vi "Create Summary Row.vi"(8 "error in (no error)":errorcluster, 10 "value":dbl, 11 "ACNET Device.lvclass":refnum<class "ACNET Device.lvclass">) -> (0 "error out":errorcluster, 3 "Summary Row":string[](array[string]))   [LabVIEW 2013, in "ACNET Monitor.lvlib"]
uses:
  ACNET Monitor.lvlib
  ACNET Device.lvclass
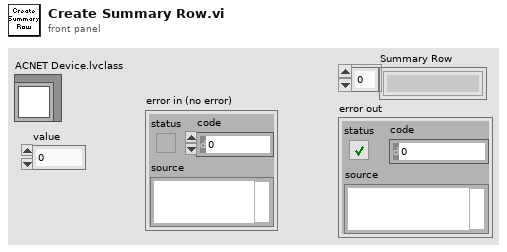
[diagram p1: front panel]
types:
  T1 = cluster{"name":string, "minValue":dbl, "maxValue":dbl, "units":string, "description":string, "ignoreMinValue":bool, "ignoreMaxValue":bool}
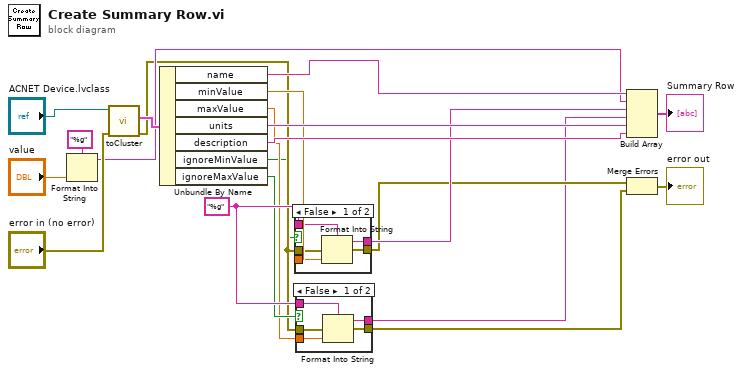
[diagram p0: block diagram]
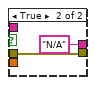
[diagram p2: hidden frame]
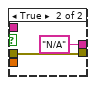
[diagram p3: hidden frame]
diagram:
  w7 = "%g" ("format string")
  n1 = Format Into String(format string="%g", "value") -> (resulting string=w11:string)  [unwired: 2 in, 1 out]
  n2 = call-dynamic "toCluster.vi"("error in (no error)"="error in (no error)", "ACNET Device in"="ACNET Device.lvclass") -> ("error out"=w5:errorcluster, "ACNET Device Cluster"=w16:T1)  [unwired: 7 in, 1 out]
  n3 = Unbundle By Name(w16) -> ("name"=w21:string, "minValue"=w17:dbl, "maxValue"=w4:dbl, "units"=w19:string, "description"=w20:string, "ignoreMinValue"=w1:bool, "ignoreMaxValue"=w6:bool)
  n4 = case shown="False" w1 {
    tunnel: [w26 "N/A"] -> w18
    tunnel: w17 -> [w25 _]
    tunnel: w5 -> [w24 w28]
    tunnel: [w23 w28] -> w9
    tunnel: w7 -> [w22 _]
    frame False {
      n5 = Format Into String(format string=w22, error in=w24, w25) -> (resulting string=w26:string, error out=w23:errorcluster)  [unwired: 1 in]
    }
    frame True {
    }
  }
  n6 = case shown="False" w6 {
    tunnel: [w33 "N/A"] -> w3
    tunnel: w4 -> [w32 _]
    tunnel: w5 -> [w31 w35]
    tunnel: [w30 w35] -> w2
    tunnel: w7 -> [w29 _]
    frame False {
      n7 = Format Into String(format string=w29, error in=w31, w32) -> (resulting string=w33:string, error out=w30:errorcluster)  [unwired: 1 in]
    }
    frame True {
    }
  }
  n8 = Build Array(w21, w11, w18, w3, w19, w20) -> (→"Summary Row":string[])
  n9 = Merge Errors(w9, w2) -> (→"error out":errorcluster)
